vi "DeadbandFilter.vi"(10 "JoystickAxis":dbl) -> (2 "FilteredJoystickAxis":dbl)   [LabVIEW 2017]
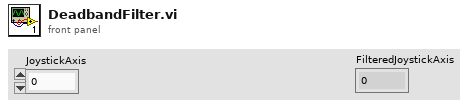
[diagram p1: front panel]
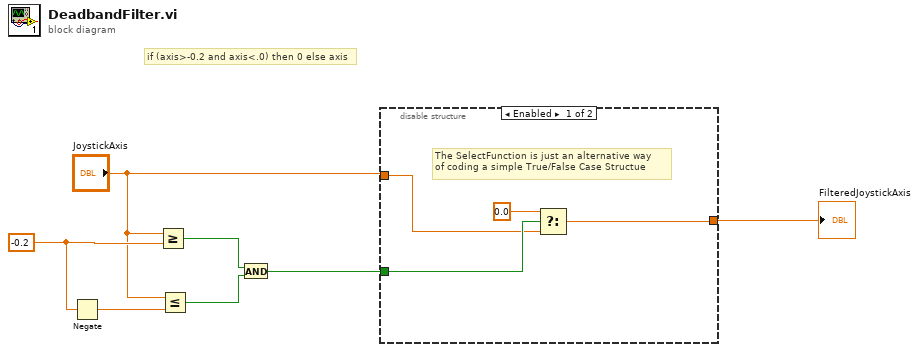
[diagram p0: block diagram]
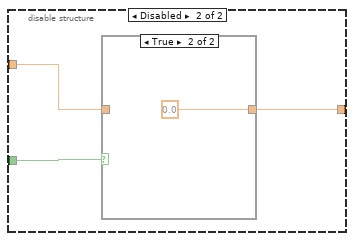
[diagram p2: hidden frame]
diagram:
  w4 = -0.2 ("y")
  # "if (axis>-0.2 and axis<.0) then 0 else axis"
  n1 = Negate(x=w4) -> (-x=w5:dbl)
  n2 = Greater Or Equal?(x="JoystickAxis", y=w4) -> (x >= y?=w6:bool)
  n3 = Less Or Equal?(x="JoystickAxis", y=w5) -> (x <= y?=w7:bool)
  n4 = And(x=w6, y=w7) -> (x .and. y?=w3:bool)
  n5 = disable-structure shown="Enabled" {
    disable-tunnel: w3 -> [w9 w14]
    disable-tunnel: "JoystickAxis" -> [w8 w13]
    disable-tunnel: [w10 w12] -> w1
    frame Enabled {
      # "The SelectFunction is just an alternative way \nof coding a simple True/False Case Structue"
      n6 = Select(t=0.0, s=w9, f=w8) -> (s? t:f=w10:dbl)
    }
    frame Disabled {
      n7 = case shown="True" w14 {
        tunnel: [w15 0.0] -> w12
        tunnel: w13 -> [w15 _]
        frame False {
        }
        frame True {
        }
      }
    }
  }
  "FilteredJoystickAxis" <- w1
